vi "OVP State inquiry.vi"(8 "error in (no error)":errorcluster, 9 "VISA resource name":refnum<visa-resource-name>, 10 "Channel  (1: CH1)":u16(ring)=1 items=["CH1"=1, "CH2"=2, "CH3"=3, "CH4"=4]) -> (0 "error out":errorcluster, 1 "VISA resource name out":refnum<visa-resource-name>, 2 "State":string)   [LabVIEW 2020, in "GPP.lvlib"]
uses:
  GPP.lvlib
  Function/VISA_COMMON.ctl
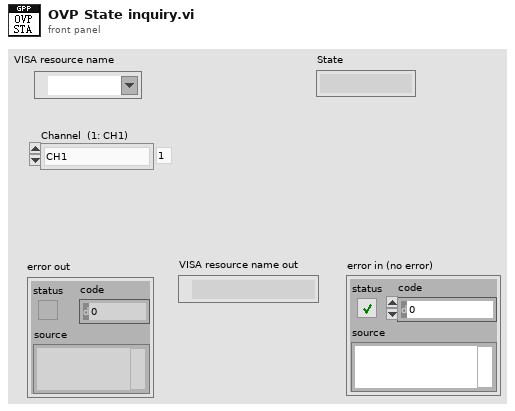
[diagram p1: front panel]
types:
  T1 = typedef "GPP.lvlib/VISA_COMMON.ctl" = enum16{"Initial", "Write CMD", "Read Result", "Read History", "Close"}
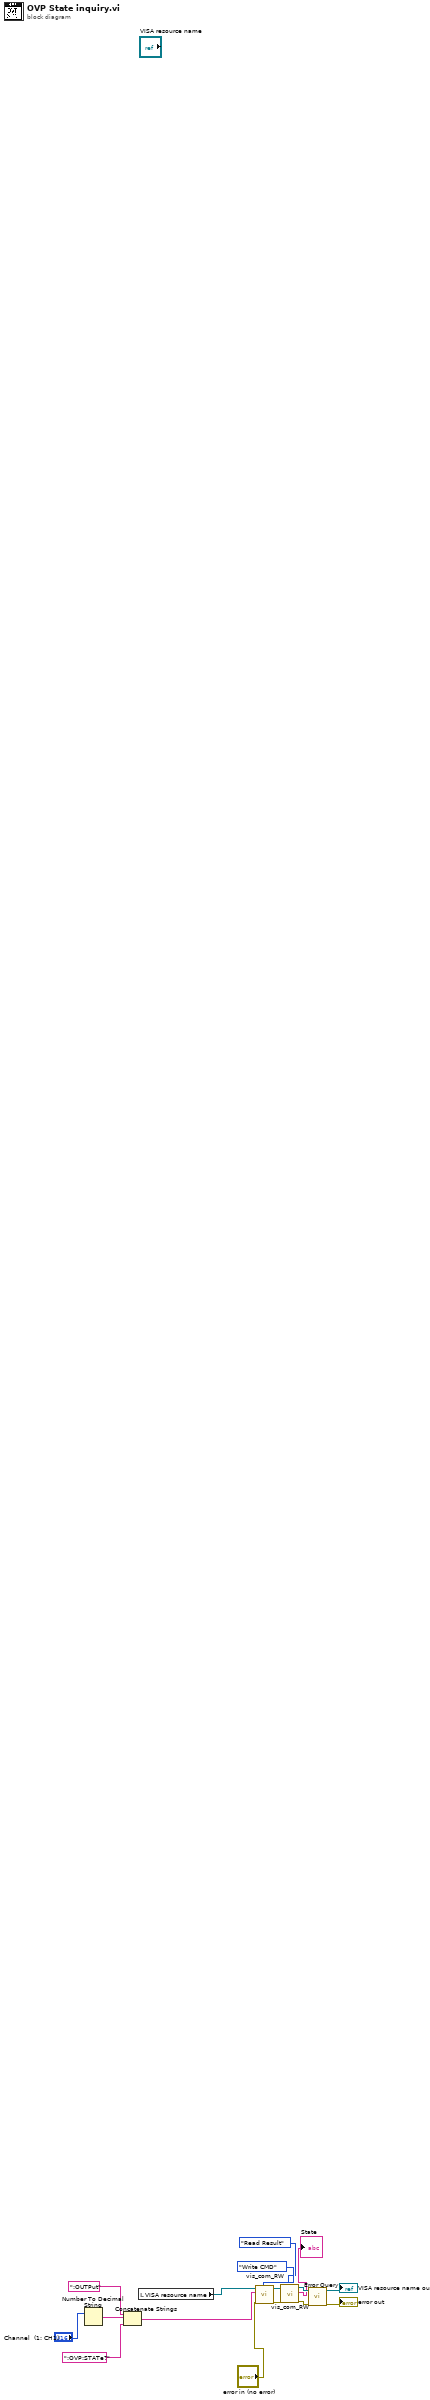
[diagram p0: block diagram]
diagram:
  n1 = Number To Decimal String(number="Channel  (1: CH1)") -> (decimal integer string=w16:string)  [unwired: 1 in]
  n2 = Concatenate Strings(":OUTPut", w16, ":OVP:STATe?") -> (w12:string)
  n3 = local read "VISA resource name"() -> (w3:refnum<visa-resource-name>)
  n4 = call "vis_com_RW.vi"("Funciton"=VISA_COMMON."Write CMD", "error in (no error)"="error in (no error)", "CMD String"=w12, "VISA resource in"=w3) -> ("error out"=w8:errorcluster, "VISA resource out"=w7:refnum<visa-resource-name>)  [unwired: 5 in, 1 out]
  n5 = call "vis_com_RW.vi"("Funciton"=VISA_COMMON."Read Result", "error in (no error)"=w8, "VISA resource in"=w7) -> ("error out"=w5:errorcluster, "Result"=→"State":string, "VISA resource out"=w6:refnum<visa-resource-name>)  [unwired: 6 in]
  n6 = call "Error Query.vi"("error in (no error)"=w5, "VISA resource name"=w6) -> ("error out"=→"error out":errorcluster, "VISA resource name out"=→"VISA resource name out":refnum<visa-resource-name>)  [unwired: 6 in, 2 out]
